vi "Test Drive fw x feet.vi"() -> ()   [LabVIEW 2017]
panel:
  out "Y-Axis":dbl
  in  "Feet":dbl
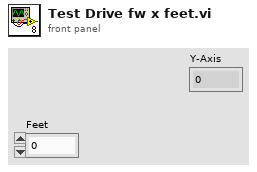
[diagram p1: front panel]
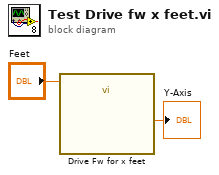
[diagram p0: block diagram]
diagram:
  n1 = call "Drive Fw for x feet.vi"("Feet"="Feet") -> ("Y-Axis"=→"Y-Axis":dbl)  [unwired: 10 in]
